vi "GDSDialog_OneButtonWindowsDialog.vi"(1 "UserText":string, 2 "ButtonName":string, 4 "Cmd":refnum<user-event>, 5 "error in (no error)":errorcluster, 6 "DialogTitle":string, 7 "TimeOutTime(ms, ignored if not wired)":i32=-1, 8 "Icon":T1(ring)=enum."Information", 9 "OK_Font:Bold(False)":bool, 10 "Text.Justification(Left)":enum16{"Left", "Center", "Right"}(ring), 11 "OK_Font:Color(Black)":u32(colorbox)) -> (15 "ButtonPressed":bool=TRUE, 16 "TimeOut":bool, 19 "error out":errorcluster)   [LabVIEW 2020]
panel:
  out "ShowIcon":T1(tab)
  out "Text":string
  in  "OK":bool
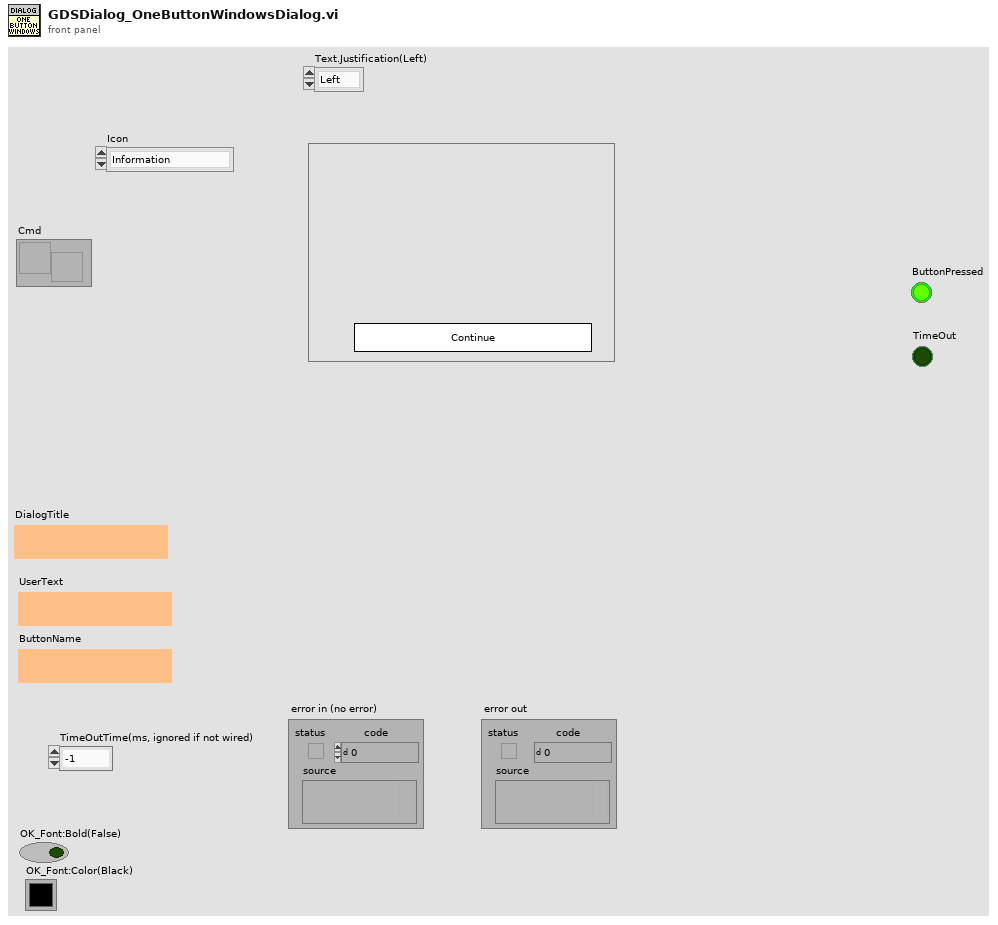
[diagram p1: front panel]
types:
  T1 = enum32{"None", "Stop", "Question", "Exclamation", "Information"}
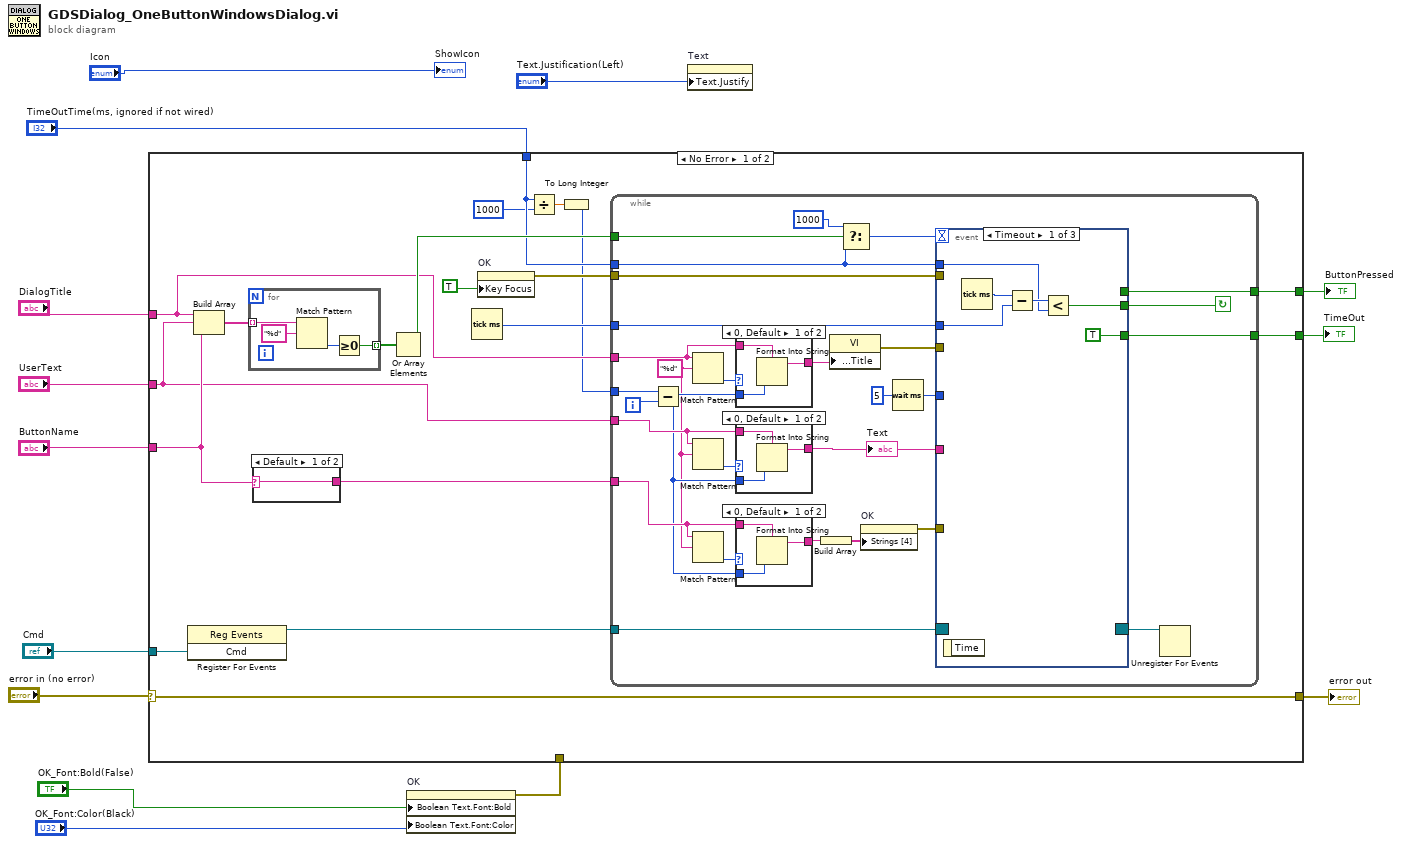
[diagram p0: block diagram]
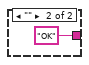
[diagram p2: hidden frame]
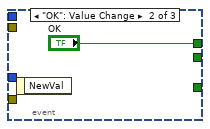
[diagram p6: hidden frame]
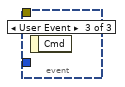
[diagram p7: hidden frame]
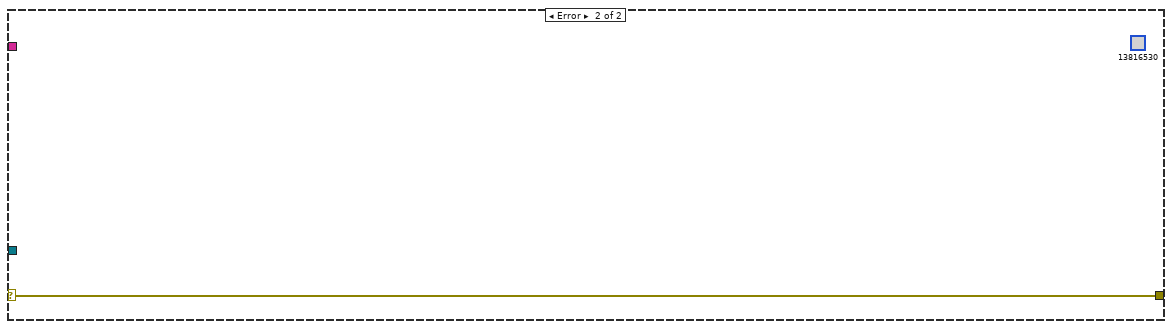
[diagram p8: hidden frame]
diagram:
  n1 = property on="OK" class="Bool"("Boolean Text.Font:Bold"="OK_Font:Bold(False)", "Boolean Text.Font:Color"="OK_Font:Color(Black)") -> (error out=w3:errorcluster)  [unwired: 2 in, 1 out]
  n2 = case shown="No Error" "error in (no error)" {
    selector: "error in (no error)" -> [w33 w88]
    tunnel: [w33 w88] -> w13
    tunnel: "UserText" -> [w19 _]
    tunnel: "DialogTitle" -> [w21 _]
    tunnel: "ButtonName" -> [w22 _]
    tunnel: "Cmd" -> [w30 _]
    tunnel: [w28 _] -> w8
    tunnel: "TimeOutTime(ms, ignored if not wired)" -> [w18 _]
    tunnel: [w27 _] -> w6
    tunnel: w3 -> [_ _]
    frame No Error {
      n3 = register-events(w30) -> (reference out=w29:refnum<event-registration>)  [unwired: 2 in, 1 out]
      n4 = Build Array(w21, w19, w22) -> (w26:string[])
      n5 = for {
        tunnel: w26 -> [w87] mode=indexing
        tunnel: [w84] -> w24 mode=indexing
        n6 = Match Pattern(string=w87, regular expression="%d") -> (offset past match=w85:i32)  [unwired: 1 in, 3 out]
        n7 = Greater Or Equal To 0?(x=w85) -> (x >= 0?=w84:bool)
      }
      n8 = case shown="Default" w22 {
        selector: w22 -> [w34 _]
        tunnel: [w34 "OK"] -> w20
        frame Default {
        }
        frame "" {
        }
      }
      n9 = Or Array Elements(Boolean array=w24) -> (logical OR=w23:bool)
      n10 = Tick Count (ms)() -> (millisecond timer value=w25:u32)
      n11 = property on="OK" class="Bool"("Key Focus"=TRUE) -> (error out=w31:errorcluster)  [unwired: 2 in, 1 out]
      n12 = Divide(x=w18, y=1000) -> (x/y=w16:dbl)
      n13 = To Long Integer(number=w16) -> (32bit integer=w15:i32)
      n14 = while {
        tunnel: w31 -> [w64]
        tunnel: w29 -> [w63]
        tunnel: [w61] -> w28
        tunnel: w18 -> [w56]
        tunnel: [w60] -> w27
        tunnel: w25 -> [w59]
        tunnel: w23 -> [w57]
        tunnel: w21 -> [w50]
        tunnel: w19 -> [w44]
        tunnel: w20 -> [w43]
        tunnel: w15 -> [w49]
        i -> [w48]
        stop <- w58 continue-if-true
        w41 = "%d" ("regular expression")
        n15 = Subtract(x=w49, y=w48) -> (x-y=w42:i32)
        n16 = Match Pattern(string=w50, regular expression=w41) -> (offset past match=w52:i32)  [unwired: 1 in, 3 out]
        n17 = Match Pattern(string=w44, regular expression=w41) -> (offset past match=w47:i32)  [unwired: 1 in, 3 out]
        n18 = Match Pattern(string=w43, regular expression=w41) -> (offset past match=w46:i32)  [unwired: 1 in, 3 out]
        n19 = case shown="0, Default" w52 {
          tunnel: [w73 w76] -> w51
          tunnel: w50 -> [w75 w76]
          tunnel: w42 -> [w74 _]
          frame 0, Default {
            n20 = Format Into String(format string=w75, w74) -> (resulting string=w73:string)  [unwired: 2 in, 1 out]
          }
          frame -1 {
          }
        }
        n21 = case shown="0, Default" w47 {
          tunnel: [w69 w72] -> w39
          tunnel: w44 -> [w71 w72]
          tunnel: w42 -> [w70 _]
          frame 0, Default {
            n22 = Format Into String(format string=w71, w70) -> (resulting string=w69:string)  [unwired: 2 in, 1 out]
          }
          frame -1 {
          }
        }
        "Text" <- w39
        n23 = case shown="0, Default" w46 {
          tunnel: [w65 w68] -> w45
          tunnel: w43 -> [w67 w68]
          tunnel: w42 -> [w66 _]
          frame 0, Default {
            n24 = Format Into String(format string=w67, w66) -> (resulting string=w65:string)  [unwired: 2 in, 1 out]
          }
          frame -1 {
          }
        }
        n25 = Build Array(w45) -> (w53:string[])
        n26 = property class="VI"("Front Panel Window:Title"=w51) -> (error out=w40:errorcluster)  [unwired: 2 in, 1 out]
        n27 = Select(t=1000, s=w57, f=w56) -> (s? t:f=w55:i32)
        n28 = property on="OK" class="Bool"("Strings [4]"=w53) -> (error out=w38:errorcluster)  [unwired: 2 in, 1 out]
        n29 = Wait (ms)(milliseconds to wait=u32 5) -> (millisecond timer value=w37:u32)
        n30 = event shown="[0] Timeout" {
          selector: w63 -> [_ _ _]
          dyn-events: [_ _ _] -> w62
          timeout: w55 -> [_ _ _]
          tunnel: w64 -> [_ _ _]
          tunnel: [_ "OK" _] -> w61
          tunnel: [TRUE _ _] -> w60
          tunnel: w59 -> [w80 _ _]
          tunnel: [w78 _ _] -> w58
          tunnel: w56 -> [w77 _ _]
          tunnel: w40 -> [_ _ _]
          tunnel: w39 -> [_ _ _]
          tunnel: w38 -> [_ _ _]
          tunnel: w37 -> [_ _ _]
          event Timeout {
            n31 = event-data() -> ()  [unwired: 1 in, 1 out]
            n32 = Tick Count (ms)() -> (millisecond timer value=w81:u32)
            n33 = Subtract(x=w81, y=w80) -> (x-y=w79:u32)
            n34 = Less?(x=w79, y=w77) -> (x < y?=w78:bool)
          }
          event "OK": Value Change {
            n35 = event-data() -> ()  [unwired: 1 in, 1 out]
          }
          event User Event {
            n36 = event-data() -> ()  [unwired: 1 in, 1 out]
          }
        }
        n37 = Unregister For Events(event registration refnum=w62) -> ()  [unwired: 1 in, 1 out]
      }
    }
    frame Error {
      (unwired) u32 13816530 ("BgColor")
    }
  }
  "error out" <- w13
  "ButtonPressed" <- w8
  "TimeOut" <- w6
  n38 = property on="Text" class="Str"("Text.Justify"="Text.Justification(Left)") -> ()  [unwired: 2 in, 2 out]
  "ShowIcon" <- "Icon"
